vi "PI (FXP).vi"(5 "Ki":fxp<+,32,8>, 7 "Kp":fxp<+,32,8>, 10 "Process Value":fxp<+/-,32,16>, 11 "Setpoint":fxp<+/-,32,16>) -> (3 "Output":fxp<+/-,32,12> format="%.24g")   [LabVIEW 2025]
uses:
  <vilib>/rvi/FXPMathLib/FxpSub/XNode/nifxpmath_Sub.xnode
  <vilib>/rvi/FXPMathLib/sim/FxpSim.dll
  <vilib>/rvi/FXPMathLib/FxpMul/XNode/nifxpmath_Multiplier.xnode
  <vilib>/rvi/FXPMathLib/FxpAdd/XNode/nifxpmath_Add.xnode
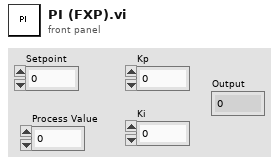
[diagram p1: front panel]
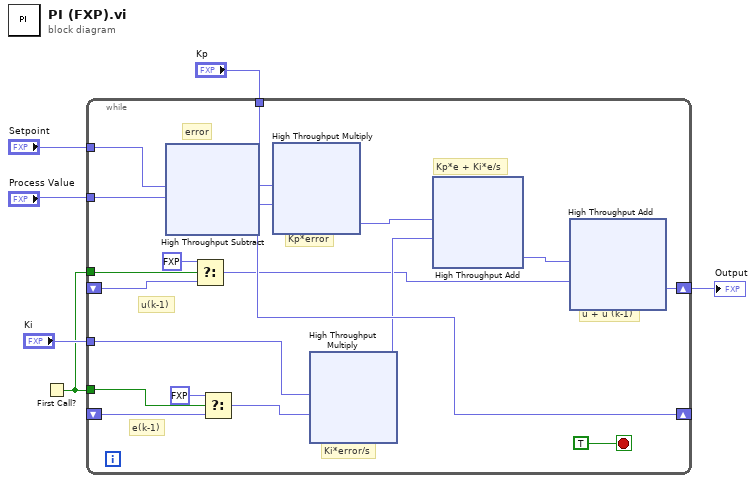
[diagram p0: block diagram]
diagram:
  n1 = First Call?() -> (First Call?: T/F=w1:bool)
  n2 = while {
    shift-right: [w22] -> _
    shift-left: _ -> [w14]
    tunnel: w1 -> [w9]
    shift-right: [w15] -> w6
    shift-left: _ -> [w16]
    tunnel: w1 -> [w19]
    tunnel: "Setpoint" -> [w13]
    tunnel: "Process Value" -> [w12]
    tunnel: "Kp" -> [w11]
    tunnel: "Ki" -> [w10]
    stop <- TRUE stop-if-true
    # "u + u (k-1)"
    # "Kp*e + Ki*e/s"
    # "Ki*error/s"
    # "Kp*error"
    # "e(k-1)"
    # "u(k-1)"
    # "error"
    n3 = xnode "High Throughput Subtract"("x"=w13, "y"=w12) -> ("x-y"=w22:fxp<+/-,32,16>)
    n4 = Select(t=fxp<+/-,32,16> 0.0, s=w19, f=w16) -> (s? t:f=w8:fxp<+/-,36,16>)
    n5 = Select(t=fxp<+/-,32,16> 0.0, s=w9, f=w14) -> (s? t:f=w21:fxp<+/-,32,16>)
    n6 = xnode "High Throughput Multiply"("x"=w11, "y"=w22) -> ("x*y"=w18:fxp<+/-,32,8>)
    n7 = xnode "High Throughput Multiply"("x"=w10, "y"=w21) -> ("x*y"=w17:fxp<+/-,32,8>)
    n8 = xnode "High Throughput Add"("x"=w18, "y"=w17) -> ("x+y"=w7:fxp<+/-,32,8>)
    n9 = xnode "High Throughput Add"("x"=w7, "y"=w8) -> ("x+y"=w15:fxp<+/-,32,12>)
  }
  "Output" <- w6
